vi "ERD_Read_Builder.vi"(5 "ERD Read List All":T1 {"ERD Number" format="%x"}, 11 "error in":errorcluster) -> (4 "Read ERD List":i32[](array[numeric]), 8 "ERD Name":string[](array[string]), 15 "error out":errorcluster)   [LabVIEW 2021]
uses:
  Controles/ERD_List.ctl
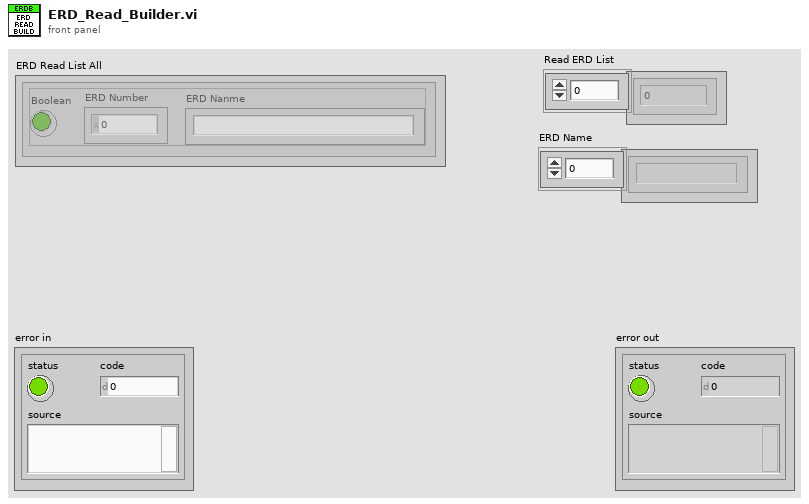
[diagram p1: front panel]
types:
  T1 = typedef "ERD_List.ctl" = cluster{"Boolean":bool, "ERD Number":i32, "ERD Nanme":string}[]
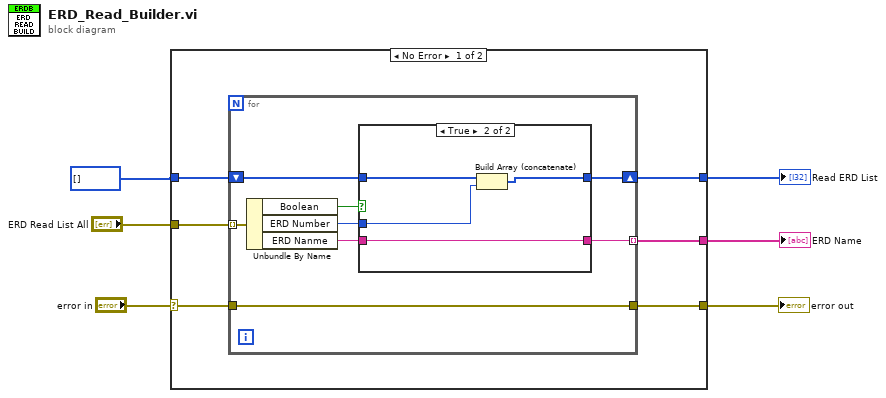
[diagram p0: block diagram]
diagram:
  n1 = case shown="No Error" "error in" {
    selector: "error in" -> [w8 w26]
    tunnel: "ERD Read List All" -> [w12 _]
    tunnel: i32[] [] ("appended array") -> [w11 _]
    tunnel: [w10 _] -> w4
    tunnel: [w9 _] -> w3
    tunnel: [w7 w26] -> w1
    frame No Error {
      n2 = for {
        tunnel: w12 -> [w20] mode=indexing
        shift-right: [w15] -> w9
        shift-left: w11 -> [w16]
        tunnel: [w14] -> w10 mode=indexing
        tunnel: w8 -> [w13]
        tunnel: [w13] -> w7
        n3 = Unbundle By Name(w20) -> ("Boolean"=w19:bool, "ERD Number"=w18:i32, "ERD Nanme"=w17:string)
        n4 = case shown="True" w19 {
          tunnel: w18 -> [_ w25]
          tunnel: w17 -> [_ w22]
          tunnel: w16 -> [w21 w24]
          tunnel: [w21 w23] -> w15
          tunnel: [_ w22] -> w14
          frame False {
          }
          frame True {
            n5 = Build Array (concatenate)(w24, w25) -> (w23:i32[])
          }
        }
      }
    }
    frame Error {
    }
  }
  "ERD Name" <- w4
  "Read ERD List" <- w3
  "error out" <- w1
